vi "Assign status from string.vi"(8 "error in (no error)":errorcluster, 9 "Read All Lines?":bool, 10 "Elements to parse":string[](array[string]), 11 "Answer to parse":string) -> (0 "error out":errorcluster, 3 "Status Array":T1[](array[typedef]))   [LabVIEW 2020]
uses:
  Status.ctl
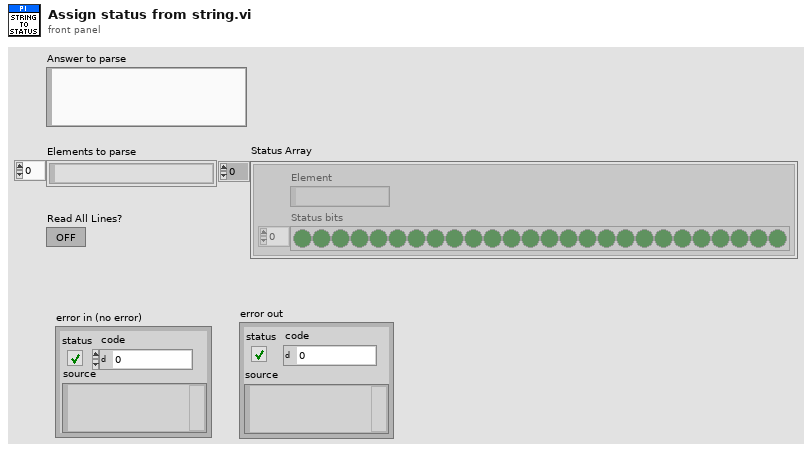
[diagram p1: front panel]
types:
  T1 = typedef "Status.ctl" = cluster{"Element":string, "Status bits":bool[]}
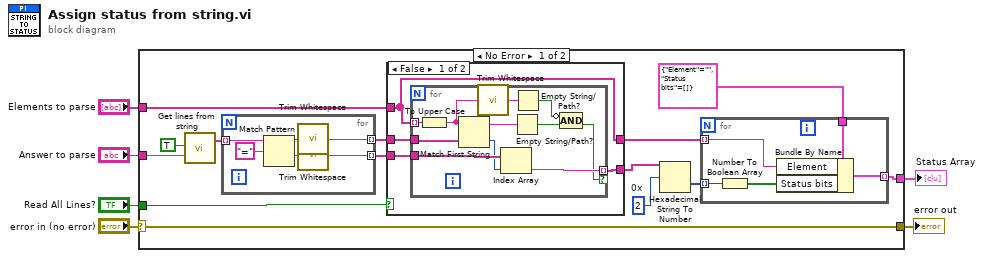
[diagram p0: block diagram]
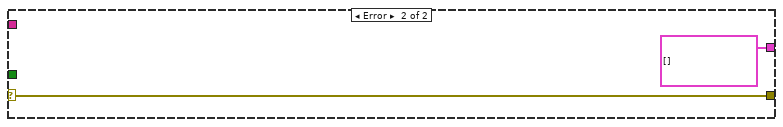
[diagram p3: hidden frame]
diagram:
  n1 = case shown="No Error" "error in (no error)" {
    selector: "error in (no error)" -> [w20 w50]
    tunnel: "Read All Lines?" -> [w16 _]
    tunnel: "Answer to parse" -> [w19 _]
    tunnel: "Elements to parse" -> [w13 _]
    tunnel: [w20 w50] -> w3
    tunnel: [w8 T1[] []] -> w1
    frame No Error {
      w7 = 2  # 0x
      n2 = call "Get lines from string.vi"("Cut spaces?"=TRUE, "Input string"=w19) -> ("Strings"=w17:string[])  [unwired: 16 in, 1 out]
      n3 = for {
        tunnel: w17 -> [w48] mode=indexing
        tunnel: [w45] -> w14 mode=indexing
        tunnel: [w43] -> w15 mode=indexing
        n4 = Match Pattern(string=w48, regular expression="=") -> (before substring=w46:string, after substring=w44:string)  [unwired: 1 in, 2 out]
        n5 = call "Trim Whitespace.vi"("string"=w46) -> ("trimmed string"=w45:string)  [unwired: 1 in]
        n6 = call "Trim Whitespace.vi"("string"=w44) -> ("trimmed string"=w43:string)  [unwired: 1 in]
      }
      n7 = case shown="False" w16 {
        tunnel: w15 -> [w28 w42]
        tunnel: w14 -> [w29 w41]
        tunnel: [w27 w42] -> w12
        tunnel: w13 -> [w26 _]
        tunnel: [w26 w41] -> w9
        frame False {
          n8 = for {
            tunnel: w26 -> [w33] mode=indexing
            tunnel: w29 -> [w40]
            tunnel: w28 -> [w39]
            tunnel: [w37] -> w27 mode=indexing if=w34
            n9 = To Upper Case(1:w33) -> (0:w30:string)
            n10 = Match First String(2:w40, 3:w30) -> (0:w38:i32, 1:w36:string)
            n11 = call "Trim Whitespace.vi"("string"=w30) -> ("trimmed string"=w32:string)  [unwired: 1 in]
            n12 = Index Array(array=w39, index=w38) -> (element=w37:string)
            n13 = Empty String/Path?(string/path=w36) -> (empty?=w35:bool)
            n14 = Empty String/Path?(string/path=w32) -> (empty?=w31:bool)
            n15 = Compound Arithmetic op=AND(invert w31, w35) -> (w34:bool)
          }
        }
        frame True {
        }
      }
      n16 = Hexadecimal String To Number(string=w12, offset=w7) -> (number=w11:u32[])  [unwired: 1 in, 1 out]
      n17 = for {
        tunnel: [w21] -> w8 mode=indexing
        tunnel: w11 -> [w25] mode=indexing
        tunnel: T1 {"Element"="", "Status bits"=[]} ("Status") -> [w24]
        tunnel: w9 -> [w22] mode=indexing
        n18 = Number To Boolean Array(number=w25) -> (Boolean array=w23:bool[])
        n19 = Bundle By Name(cluster=w24, "Element"=w22, "Status bits"=w23) -> (w21:T1)
      }
    }
    frame Error {
    }
  }
  "error out" <- w3
  "Status Array" <- w1
